vi "Aim_Turret_with_Camera.vi"(8 "Change Angles":bool, 10 "Angle Change":dbl=10.0, 11 "Current Encoder Pos":dbl) -> (3 "New Encoder Pos":dbl)   [LabVIEW 2012]
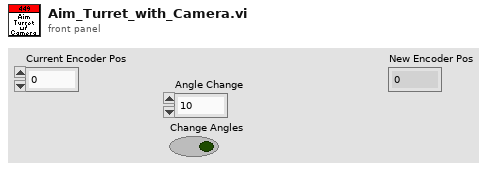
[diagram p1: front panel]
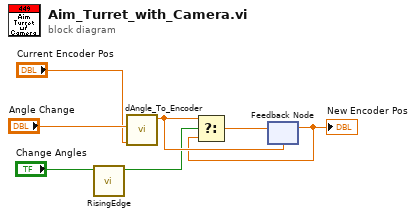
[diagram p0: block diagram]
diagram:
  n1 = call "RisingEdge.vi"("BooleanIn"="Change Angles") -> ("BooleanOut"=w3:bool)  [unwired: 10 in]
  n2 = call "dAngle_To_Encoder.vi"("Current Encoder Pos"="Current Encoder Pos", "Angle Change"="Angle Change") -> ("New Encoder Pos"=w4:dbl)  [unwired: 9 in]
  n3 = feedback #1(w4) -> (w1:dbl)
  "New Encoder Pos" <- w1
  n4 = Select(t=w4, s=w3, f=w1) -> (s? t:f=w5:dbl)
  n5 = feedback-in #1(w5) -> ()
